vi "CAL-Daten speichern.vi"(0 "CAL-Daten PMA":T4={"O2 Null"=0.0, "O2 Steil"=[1.0, 1.0, 1.0, 1.0]}, 1 "CAL-Daten FID":T1={"CH4 Null"=0.0, "CH4 Steil"=[1.0, 1.0, 1.0, 1.0], "THC Null"=0.0, "THC Steil"=[1.0, 1.0, 1.0, 1.0], "NMHC Null"=0.0, "NMHC Steil"=[1.0, 1.0, 1.0, 1.0]}, 2 "Polynom":sgl[][](array[numeric]), 3 "Aktiv":bool[](array[boolean]), 4 "CAL-Daten Tolernaz":T2, 11 "Aktionen Kal Daten speichern":T3) -> ()   [LabVIEW 2020, in "ABB-EL3000.lvlib" / "Allgemeine VI.lvlib"]
uses:
  Allgemeine VI.lvlib
  CAL-Daten PMA.ctl
  Aktionen Cal Daten speichern.ctl
  CAL-Daten Toleranz.ctl
  CAL-Daten FID.ctl
  <vilib>/Utility/config.llb/Write Key (String).vi
  <vilib>/Utility/config.llb/NI_LVConfig.lvlib
  Allgemein/allgemeine Sub-VIs.lvlib
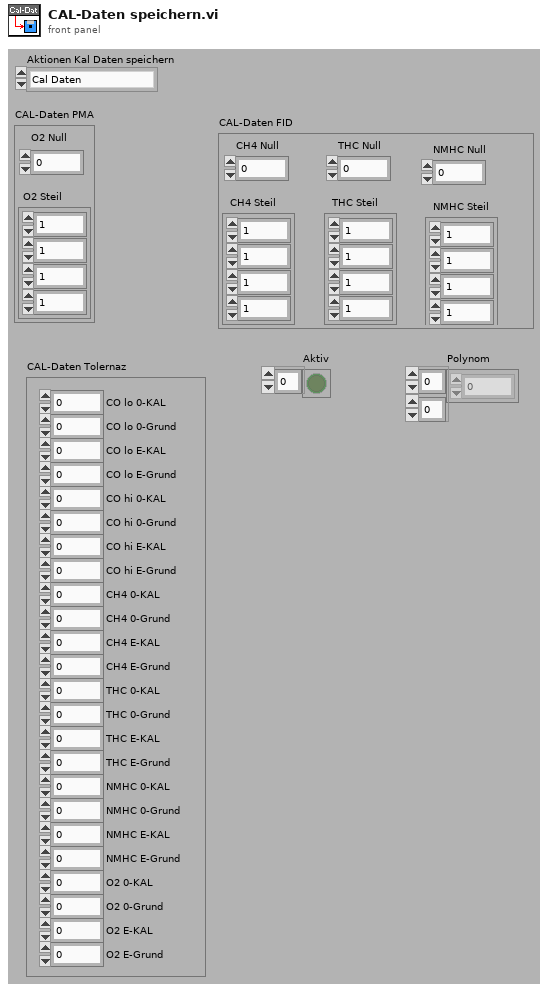
[diagram p1: front panel]
types:
  T1 = typedef "ABB-EL3000.lvlib/Allgemeine VI.lvlib/CAL-Daten FID.ctl" = cluster{"CH4 Null":sgl, "CH4 Steil":sgl[], "THC Null":sgl, "THC Steil":sgl[], "NMHC Null":sgl, "NMHC Steil":sgl[]}
  T2 = typedef "ABB-EL3000.lvlib/Allgemeine VI.lvlib/CAL-Daten Toleranz.ctl" = cluster{"CO lo 0-KAL":sgl, "CO lo 0-Grund":sgl, "CO lo E-KAL":sgl, "CO lo E-Grund":sgl, "CO hi 0-KAL":sgl, "CO hi 0-Grund":sgl, "CO hi E-KAL":sgl, "CO hi E-Grund":sgl, "CH4 0-KAL":sgl, "CH4 0-Grund":sgl, "CH4 E-KAL":sgl, "CH4 E-Grund":sgl, "THC 0-KAL":sgl, "THC 0-Grund":sgl, "THC E-KAL":sgl, "THC E-Grund":sgl, "NMHC 0-KAL":sgl, "NMHC 0-Grund":sgl, "NMHC E-KAL":sgl, "NMHC E-Grund":sgl, "O2 0-KAL":sgl, "O2 0-Grund":sgl, "O2 E-KAL":sgl, "O2 E-Grund":sgl}
  T3 = typedef "ABB-EL3000.lvlib/Allgemeine VI.lvlib/Aktionen Cal Daten speichern.ctl" = enum16{"Cal Daten", "Toleranzen", "PMA", "FID", "Cal Daten PMA", "Cal Daten FID"}
  T4 = typedef "ABB-EL3000.lvlib/Allgemeine VI.lvlib/CAL-Daten PMA.ctl" = cluster{"O2 Null":sgl, "O2 Steil":sgl[]}
  T5 = typedef "NI_LVConfig.lvlib/Config Data RefNum.ctl" = refnum<k1>
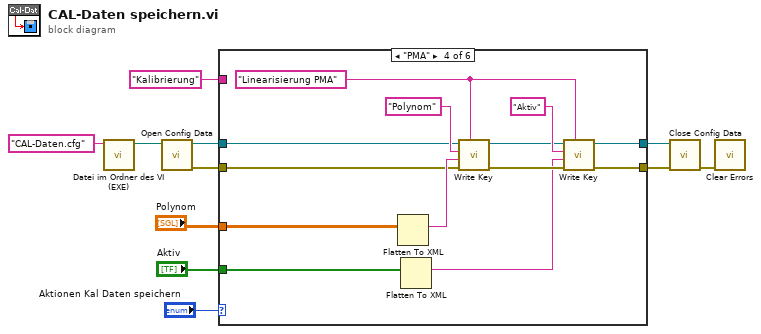
[diagram p0: block diagram]
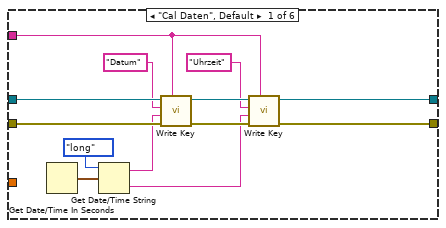
[diagram p2: hidden frame]
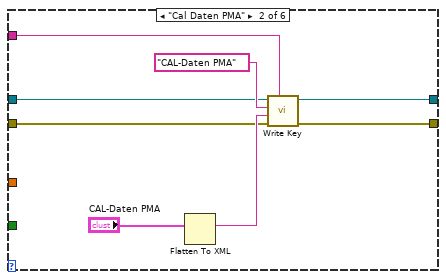
[diagram p3: hidden frame]
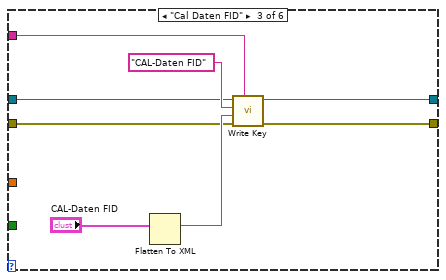
[diagram p4: hidden frame]
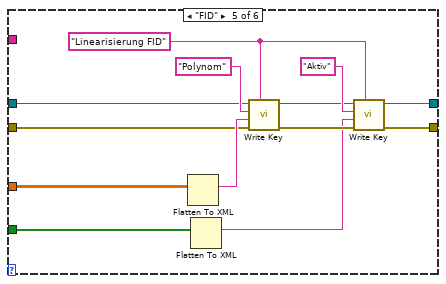
[diagram p5: hidden frame]
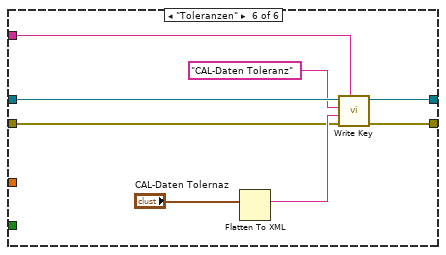
[diagram p6: hidden frame]
diagram:
  n1 = call "Datei im Ordner des VI (EXE).vi"("Dateiname"="CAL-Daten.cfg") -> ("Dateipfad im Ordner des Haupt-VIs"=w10:path)  [unwired: 8 in, 2 out]
  n2 = call <vilib>:"Open Config Data.vi"("configuration file path"=w10) -> ("error out"=w6:errorcluster, "refnum"=w7:T5)  [unwired: 8 in, 1 out]
  n3 = case shown="\"PMA\"" "Aktionen Kal Daten speichern" {
    tunnel: [w12 w29 w37 w48 w61 w71] -> w9
    tunnel: [w13 w28 w36 w47 w60 w70] -> w8
    tunnel: w7 -> [w24 w27 w35 w44 w57 w73]
    tunnel: w6 -> [w23 w26 w34 w43 w56 w72]
    tunnel: "Kalibrierung" ("section") -> [w14 w30 w38 _ _ w68]
    tunnel: "Polynom" -> [_ _ _ w42 w55 _]
    tunnel: "Aktiv" -> [_ _ _ w41 w54 _]
    frame "Cal Daten", Default {
      n4 = Get Date/Time In Seconds() -> (seconds since 1Jan1904=w21:timestamp)
      n5 = Get Date/Time String(date format (0)=enum16{"short", "long", "abbreviated"}."long" ("Datumsformat (0)"), seconds (now)=w21) -> (date string=w15:string, time string=w16:string)  [unwired: 1 in]
      n6 = call-poly <vilib>:"Write Key.vi"("section"=w14, "error in (no error)"=w23, "value"=w15, "key"="Datum", "refnum"=w24) -> ("error out"=w18:errorcluster, "refnum out"=w19:T5)  [unwired: 1 in, 4 out]
      n7 = call-poly <vilib>:"Write Key.vi"("section"=w14, "error in (no error)"=w18, "value"=w16, "key"="Uhrzeit", "refnum"=w19) -> ("error out"=w13:errorcluster, "refnum out"=w12:T5)  [unwired: 1 in, 4 out]
    }
    frame "Cal Daten PMA" {
      n8 = Flatten To XML(6:"CAL-Daten PMA") -> (2:w31:string)
      n9 = call-poly <vilib>:"Write Key.vi"("section"=w30, "error in (no error)"=w26, "value"=w31, "key"="CAL-Daten PMA", "refnum"=w27) -> ("error out"=w28:errorcluster, "refnum out"=w29:T5)  [unwired: 1 in, 4 out]
    }
    frame "Cal Daten FID" {
      n10 = Flatten To XML(6:"CAL-Daten FID") -> (2:w39:string)
      n11 = call-poly <vilib>:"Write Key.vi"("section"=w38, "error in (no error)"=w34, "value"=w39, "key"="CAL-Daten FID", "refnum"=w35) -> ("error out"=w36:errorcluster, "refnum out"=w37:T5)  [unwired: 1 in, 4 out]
    }
    frame "PMA" {
      w45 = "Linearisierung PMA" ("key")
      n12 = Flatten To XML(6:w42) -> (2:w46:string)
      n13 = Flatten To XML(6:w41) -> (2:w49:string)
      n14 = call-poly <vilib>:"Write Key.vi"("section"=w45, "error in (no error)"=w43, "value"=w46, "key"="Polynom", "refnum"=w44) -> ("error out"=w51:errorcluster, "refnum out"=w52:T5)  [unwired: 1 in, 4 out]
      n15 = call-poly <vilib>:"Write Key.vi"("section"=w45, "error in (no error)"=w51, "value"=w49, "key"="Aktiv", "refnum"=w52) -> ("error out"=w47:errorcluster, "refnum out"=w48:T5)  [unwired: 1 in, 4 out]
    }
    frame "FID" {
      w58 = "Linearisierung FID" ("key")
      n16 = Flatten To XML(6:w55) -> (2:w59:string)
      n17 = Flatten To XML(6:w54) -> (2:w62:string)
      n18 = call-poly <vilib>:"Write Key.vi"("section"=w58, "error in (no error)"=w56, "value"=w59, "key"="Polynom", "refnum"=w57) -> ("error out"=w64:errorcluster, "refnum out"=w65:T5)  [unwired: 1 in, 4 out]
      n19 = call-poly <vilib>:"Write Key.vi"("section"=w58, "error in (no error)"=w64, "value"=w62, "key"="Aktiv", "refnum"=w65) -> ("error out"=w60:errorcluster, "refnum out"=w61:T5)  [unwired: 1 in, 4 out]
    }
    frame "Toleranzen" {
      n20 = Flatten To XML(6:"CAL-Daten Tolernaz") -> (2:w74:string)
      n21 = call-poly <vilib>:"Write Key.vi"("section"=w68, "error in (no error)"=w72, "value"=w74, "key"="CAL-Daten Toleranz", "refnum"=w73) -> ("error out"=w70:errorcluster, "refnum out"=w71:T5)  [unwired: 1 in, 4 out]
    }
  }
  n22 = call <vilib>:"Close Config Data.vi"("error in (no error)"=w8, "refnum"=w9) -> ("error out"=w3:errorcluster)  [unwired: 1 in, 8 out]
  n23 = call <vilib>:"Clear Errors.vi"("error in (no error)"=w3) -> ()  [unwired: 5 in, 2 out]
